vi "FGV Zustaende.vi"(6 "Aktionen":T4, 7 "SL SV Cluster":T2, 8 "Samplepoint":u16, 9 "aktuelle Bildnummer":T1=enum."Grafik", 10 "Zustand cRIO":T3, 11 "Zustand PC":T3) -> (0 "Samplepoint":u16, 1 "aktuelle Bildnummer":T1, 2 "Zustand cRIO":T3, 3 "Zustand PC":T3, 5 "SL SV Cluster":T2)   [LabVIEW 2020, in "Allgemein.lvlib"]
uses:
  Allgemein.lvlib
  Funktionstasten/Zustaende.ctl
  FGV Zustaende Aktionen.ctl
  Bildwechsel/Bild-Auswahl.ctl
  Funktionstasten/Funktionstasten.lvlib
  Bildwechsel/Bildwechsel.lvlib
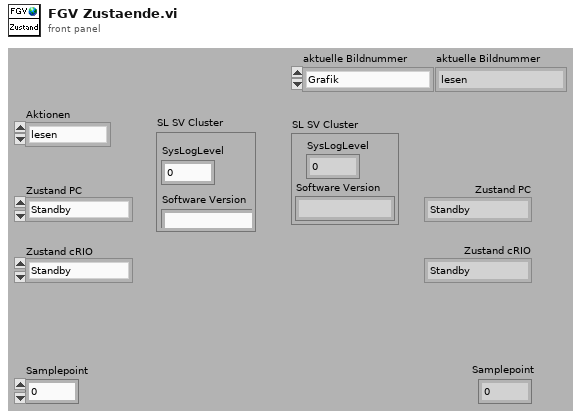
[diagram p1: front panel]
types:
  T1 = typedef "Bildwechsel.lvlib/Bild-Auswahl.ctl" = enum16{"lesen", "Initialisieren", "Beenden", "Grafik", "Anlagenübersicht", "Anlagengrenzwerte", "Log Konfig", "Gaszuordnung AO", "Erw. Konfiguration", "FT-IR  ", "Störmeldungen", "Störmeldepuffer", "Störmeldekonfig", "PNS Grenzwerte", "Statusübersicht", "Linearisierung", "ARN", "EPA Dichtheitstest", "FID", "PMA", "CalGas", "Lambda", "Interference", "Amium PNS", "EPA T90", "Interference N2O", "Scheduler", "Systemeinstellungen", "EPA Drift", "CAN Konfig"}
  T2 = cluster{"SysLogLevel":u16, "Software Version":string}
  T3 = typedef "Funktionstasten.lvlib/Zustaende.ctl" = enum16{"Standby", "Pause", "Eco", "Messen", "Kalibrieren", "Spülen Filter", "Spülen Leitung", "Umgebungsluft", "0-Gas", "Cal-Gas", "CG zu PNS", "-------------", "Init 1", "Init 2", "Init 3", "Init 4", "Messen vorbereiten", "Messen durchführen", "Exit"}
  T4 = typedef "Allgemein.lvlib/FGV Zustaende Aktionen.ctl" = enum16{"lesen", "Zustand PC", "Zustand cRIO", "Bildnummer", "Samplepoint", "Sysloglevel"}
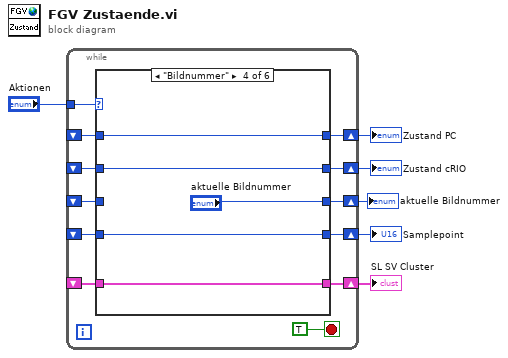
[diagram p0: block diagram]
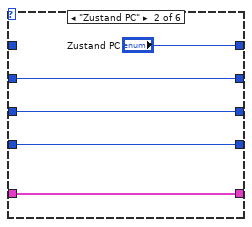
[diagram p3: hidden frame]
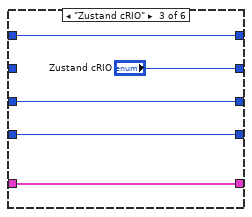
[diagram p4: hidden frame]
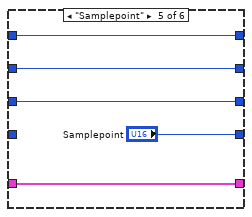
[diagram p5: hidden frame]
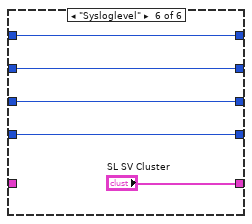
[diagram p6: hidden frame]
diagram:
  n1 = while {
    tunnel: "Aktionen" -> [w17]
    shift-right: [w15] -> w5
    shift-left: _ -> [w16]
    shift-right: [w13] -> w4
    shift-left: _ -> [w14]
    shift-right: [w11] -> w1
    shift-left: _ -> [w12]
    shift-right: [w9] -> w3
    shift-left: _ -> [w10]
    shift-right: [w8] -> w2
    shift-left: _ -> [w7]
    stop <- TRUE stop-if-true
    n2 = case shown="\"Bildnummer\"" w17 {
      tunnel: w16 -> [w23 _ w33 w38 w43 w44]
      tunnel: [w23 "Zustand PC" w33 w38 w43 w44] -> w15
      tunnel: w14 -> [w22 w27 _ w37 w42 w45]
      tunnel: [w22 w27 "Zustand cRIO" w37 w42 w45] -> w13
      tunnel: w12 -> [w21 w26 w32 _ w41 w46]
      tunnel: [w21 w26 w32 "aktuelle Bildnummer" w41 w46] -> w11
      tunnel: w10 -> [w20 w25 w31 w36 _ w47]
      tunnel: [w20 w25 w31 w36 "Samplepoint" w47] -> w9
      tunnel: [w19 w24 w29 w35 w39 "SL SV Cluster"] -> w8
      tunnel: w7 -> [w19 w24 w29 w35 w39 _]
      frame "lesen", Default {
      }
      frame "Zustand PC" {
      }
      frame "Zustand cRIO" {
      }
      frame "Bildnummer" {
      }
      frame "Samplepoint" {
      }
      frame "Sysloglevel" {
      }
    }
  }
  "Zustand PC" <- w5
  "Zustand cRIO" <- w4
  "Samplepoint" <- w3
  "SL SV Cluster" <- w2
  "aktuelle Bildnummer" <- w1
